vi "Alias Not Found--error.vi"() -> (2 "Error":errorcluster)   [LabVIEW 2020, in "jettl.lvlib" / "Error.lvlib"]
uses:
  Error.lvlib
  Actor/Actor.lvlib
  Actor/--X.ctl
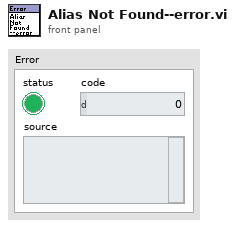
[diagram p1: front panel]
types:
  T1 = typedef "jettl.lvlib/Actor.lvlib/--X.ctl" = enum16{"--alias", "--create", "--error"}
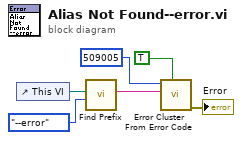
[diagram p0: block diagram]
diagram:
  n1 = control-ref of="This VI"() -> (w5:refnum<vi>)
  n2 = call "Find Prefix.vi"("--X"=--X."--error", "VI Ref"=w5) -> ("Prefix"=w3:string)  [unwired: 9 in]
  n3 = call <vilib>:"Error Cluster From Error Code.vi"("show call chain? (False)"=TRUE, "error message (\"\")"=w3, "error code (0)"=509005) -> ("error out"=→"Error":errorcluster)  [unwired: 6 in]
